vi "Read_Class_Power_Supply.vi"(8 "error in (no error)":errorcluster caption="entrée d'erreur (pas d'erreur)", 11 "Class Instrument Multimeter en entrée":refnum<class "Class Instrument Power_Supply.lvclass">) -> (0 "error out":errorcluster caption="sortie d'erreur", 2 "Power_Supply (Default)":refnum<class "Power_Supply (Default).lvclass">, 3 "Class Instrument Multimeter en sortie":refnum<class "Class Instrument Power_Supply.lvclass">)   [LabVIEW 2020, in "Library Instrument & Equipement.lvlib" / "Library Instruments.lvlib" / "Class Instrument Power_Supply.lvclass"]
uses:
  Class Instrument Power_Supply.lvclass
  Power_Supply/Power_Supply (Default)/Power_Supply (Default).lvclass
  Class Instrument Power_Supply.lvclass/Class Instrument Power_Supply.ctl
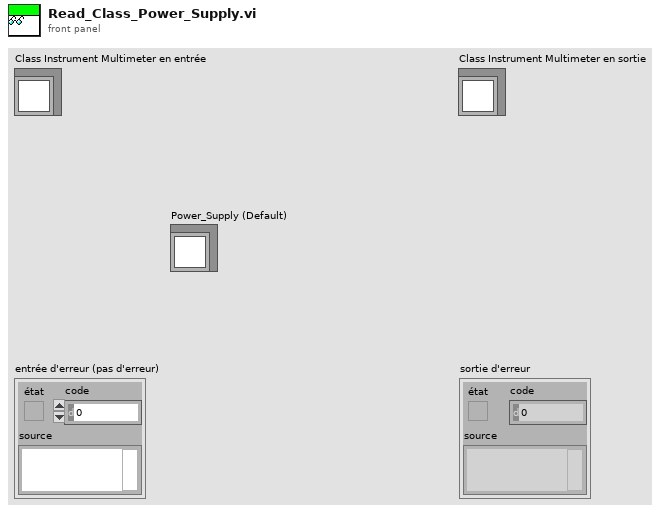
[diagram p1: front panel]
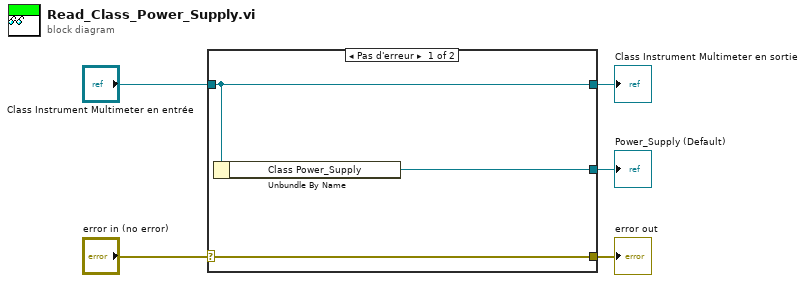
[diagram p0: block diagram]
diagram:
  n1 = case shown="Pas d'erreur" "error in (no error)" {
    selector: "error in (no error)" -> [w8 w9]
    tunnel: [w8 w9] -> w4
    tunnel: [w7 w10] -> w2
    tunnel: "Class Instrument Multimeter en entrée" -> [w7 w10]
    tunnel: [w6 _] -> w1
    frame No Error {
      n2 = Unbundle By Name(w7) -> ("Class Power_Supply"=w6:refnum<class "Power_Supply (Default).lvclass">)
    }
    frame Error {
    }
  }
  "error out" <- w4
  "Class Instrument Multimeter en sortie" <- w2
  "Power_Supply (Default)" <- w1
